vi "Remove Subscriber.vi"(8 "error in (no error)":errorcluster, 10 "Topic Name":string, 11 "Topic Actor in":refnum<class "Topic Actor.lvclass">) -> (0 "error out":errorcluster, 3 "Topic Actor out":refnum<class "Topic Actor.lvclass">)   [LabVIEW 2016, in "Stream Mediator.lvlib" / "Topic Actor.lvclass"]
doc: "--\nCopyright © 2017 Composed SystemsI All rights reserved.\n\nAuthor: Jon McBee <jon.mcbee@composed.io>\n\nThis library is provided \"AS IS\" ,WITHOUT WARRANTIES OR\nCONDITIONS OF ANY KIND, either express or implied.\n\nComposed Systems -- composed.io\n\nStream 0.0.1.1\nJon McBee - Composed Systems\nCopyright (c) 2017, Composed Systems"
uses:
  <userlib>/Composed Systems/Stream/Mediator/Classes/Topic Actor/Topic Actor.lvclass
  <userlib>/Composed Systems/Stream/Mediator/Classes/Topic Actor/Topic Actor.lvclass/Topic Actor.ctl
  <userlib>/Composed Systems/Stream/Mediator/Classes/Subscriber Look Up Table/Subscriber Look Up Table.lvclass
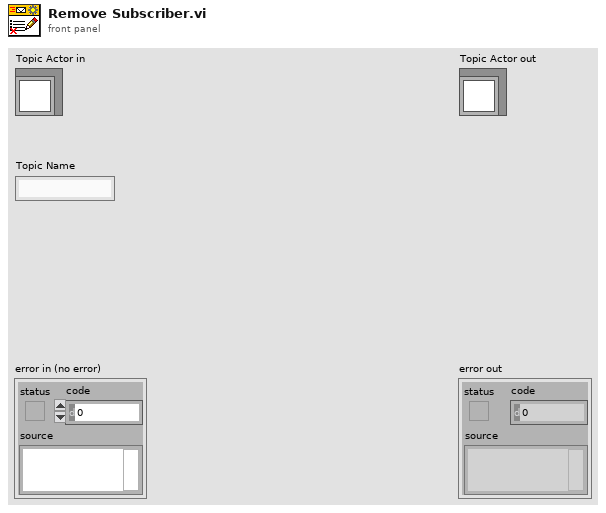
[diagram p1: front panel]
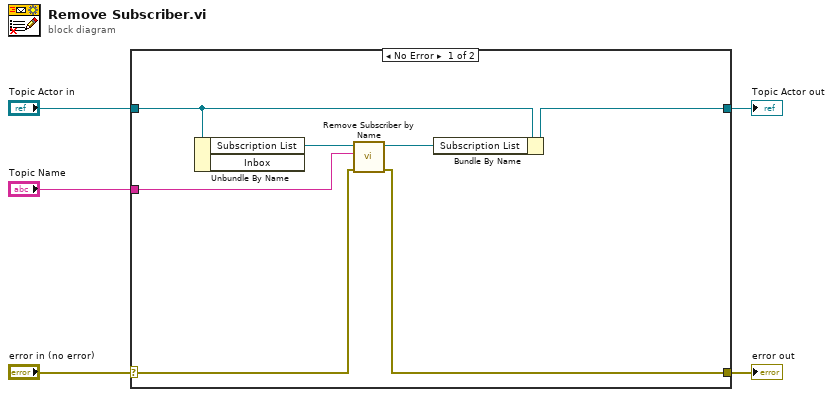
[diagram p0: block diagram]
diagram:
  n1 = case shown="No Error" "error in (no error)" {
    selector: "error in (no error)" -> [w8 w14]
    tunnel: [w7 w14] -> w4
    tunnel: [w10 w13] -> w2
    tunnel: "Topic Actor in" -> [w11 w13]
    tunnel: "Topic Name" -> [w9 _]
    frame No Error {
      n2 = Unbundle By Name(w11) -> ("Subscription List"=w12:refnum<class "Subscriber Look Up Table.lvclass">)  [unwired: 1 out]
      n3 = call <userlib>:"Remove Subscriber by Name.vi"("error in (no error)"=w8, "Topic Name"=w9, "Subscriber Look Up Table in"=w12) -> ("error out"=w7:errorcluster, "Subscriber Look Up Table out"=w6:refnum<class "Subscriber Look Up Table.lvclass">)  [unwired: 6 in, 1 out]
      n4 = Bundle By Name(cluster=w11, "Subscription List"=w6) -> (w10:refnum<class "Topic Actor.lvclass">)
    }
    frame Error {
    }
  }
  "error out" <- w4
  "Topic Actor out" <- w2
